vi "LSX Set Corr Tbl On.vi"(8 "error in (no error)":errorcluster, 10 "pcAFileName":string, 11 "lLSID":i32) -> (0 "error out":errorcluster, 2 "pcAFileName out":string, 3 "function return":i32)   [LabVIEW 2018, in "Tango.lvlib"]
doc: "TANGOAPI int TANGOCALL LSX_SetCorrTblOn (int lLSID, char *pcAFileName);"
uses:
  <userlib>/Tango/Tango.lvlib
  <userlib>/Tango/Tango_DLL.dll
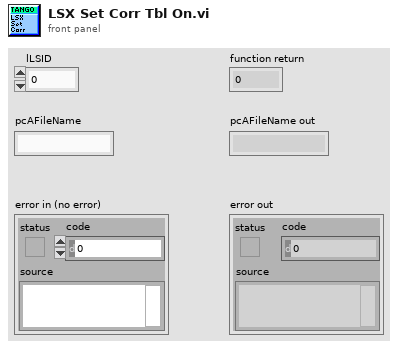
[diagram p1: front panel]
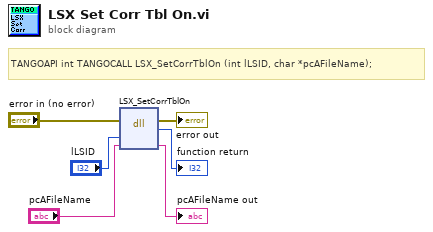
[diagram p0: block diagram]
diagram:
  # "TANGOAPI int TANGOCALL LSX_SetCorrTblOn (int lLSID, char *pcAFileName);"
  n1 = dll-call lib="C:/Program Files (x86)/National Instruments/LabVIEW 2018/user.lib/Tango/Tango_DLL.*" fn="LSX_SetCorrTblOn"(error in="error in (no error)", "lLSID"="lLSID", "pcAFileName"="pcAFileName") -> (error out=→"error out":errorcluster, →"function return":i32, "pcAFileName"=→"pcAFileName out":string)  [unwired: 3 in, 1 out]
